vi "Access Token.vi"(11 "Authorization in":refnum<class "Authorization.lvclass">) -> (2 "Access Token":string)   [LabVIEW 2020, in "OAuth2.lvlib" / "Authorization.lvclass"]
doc: "If the Authorization is valid then this returns the bearer token that should be used with requests to the desired APIs."
uses:
  Authorization.lvclass
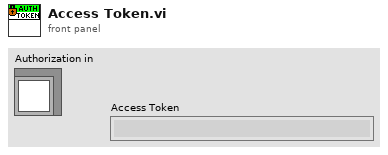
[diagram p1: front panel]
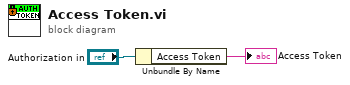
[diagram p0: block diagram]
diagram:
  n1 = Unbundle By Name("Authorization in") -> ("Access Token"=→"Access Token":string)
